vi "Self-Test.vi"(0 "VISA resource name":refnum<visa-resource-name>, 11 "error in (no error)":errorcluster) -> (4 "VISA resource name out":refnum<visa-resource-name>, 8 "Self-Test Error":u32, 10 "Self-Test Response":string, 15 "error out":errorcluster)   [LabVIEW 2015, in "Chroma ATE 6310.lvlib"]
doc: "This VI causes the instrument to perform a self-test and returns the results. This Instrument does not support a self-test and this VI will return a warning code if it is executed."
uses:
  <instrlib>/Chroma ATE 6310/Chroma ATE 6310.lvlib
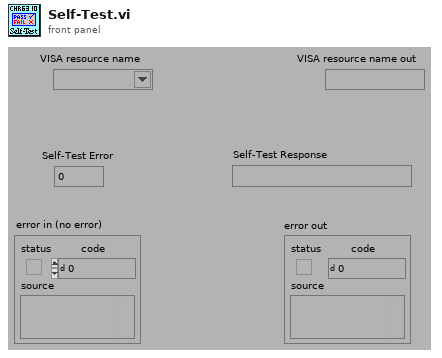
[diagram p1: front panel]
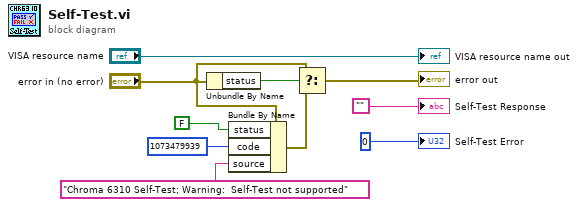
[diagram p0: block diagram]
diagram:
  n1 = Unbundle By Name("error in (no error)") -> ("status"=w4:bool)
  n2 = Bundle By Name(cluster="error in (no error)", "status"=FALSE, "code"=1073479939, "source"="Chroma 6310 Self-Test; Warning:  Self-Test not supported") -> (w5:errorcluster)
  n3 = Select(t="error in (no error)", s=w4, f=w5) -> (s? t:f=→"error out":errorcluster)
  "Self-Test Response" <- ""
  "Self-Test Error" <- u32 0
  "VISA resource name out" <- "VISA resource name"
